vi "ReadResults.vi"() -> ()   [LabVIEW 2014]
uses:
  <vilib>/xml/Load XML File.vi
  <vilib>/xml/Close Reference(Node).vi
  <vilib>/xml/NI_XML.lvlib
panel:
  out "Array":string[][](array[string])
  in  "XPath expression":string
  in  "Path":path
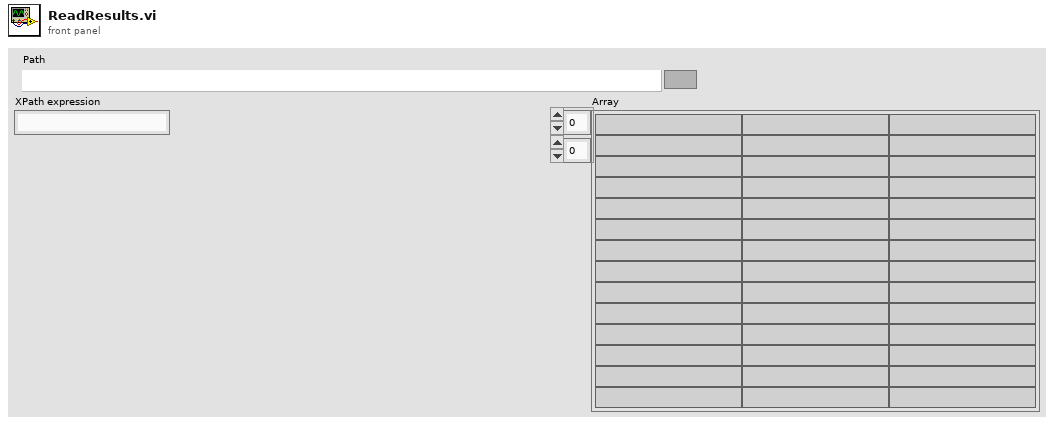
[diagram p1: front panel]
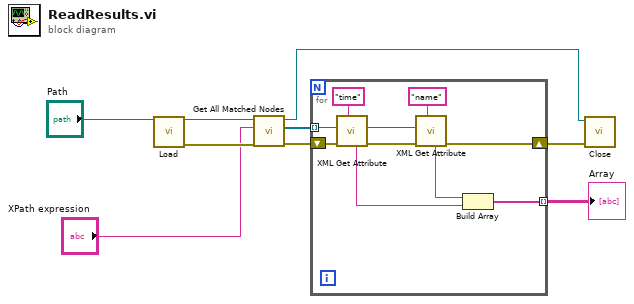
[diagram p0: block diagram]
diagram:
  n1 = call-poly <vilib>:"Load.vi"("path to XML document"="Path") -> ("DOM document out"=w8:refnum<k20>, "error out"=w7:errorcluster)  [unwired: 12 in, 1 out]
  n2 = call <vilib>:"Get All Matched Nodes.vi"("error in (no error)"=w7, "XPath expression"="XPath expression", "node in"=w8) -> ("error out"=w4:errorcluster, "node result array"=w5:refnum<k20>[], "node out"=w2:refnum<k20>)  [unwired: 6 in]
  n3 = for {
    tunnel: w5 -> [w17] mode=indexing
    shift-right: [w10] -> w3
    shift-left: w4 -> [w18]
    tunnel: [w19] -> w1 mode=indexing
    n4 = call "XML Get Attribute.vi"("attribute"="time", "error in"=w18, "node in"=w17) -> ("error out"=w14:errorcluster, "node out"=w15:refnum<k20>, "value"=w13:string)  [unwired: 4 in]
    n5 = call "XML Get Attribute.vi"("attribute"="name" ("XPath expression"), "error in"=w14, "node in"=w15) -> ("error out"=w10:errorcluster, "value"=w12:string)  [unwired: 4 in, 1 out]
    n6 = Build Array(w12, w13) -> (w19:string[])
  }
  "Array" <- w1
  n7 = call-poly <vilib>:"Close.vi"("error in (no error)"=w3, "node"=w2) -> ()  [unwired: 7 in, 1 out]
